vi "数据库存储.vi"(3 "输出簇":T1) -> ()   [LabVIEW 2010]
panel:
  in  "error in (no error)":errorcluster caption="错误输入（无错误）"
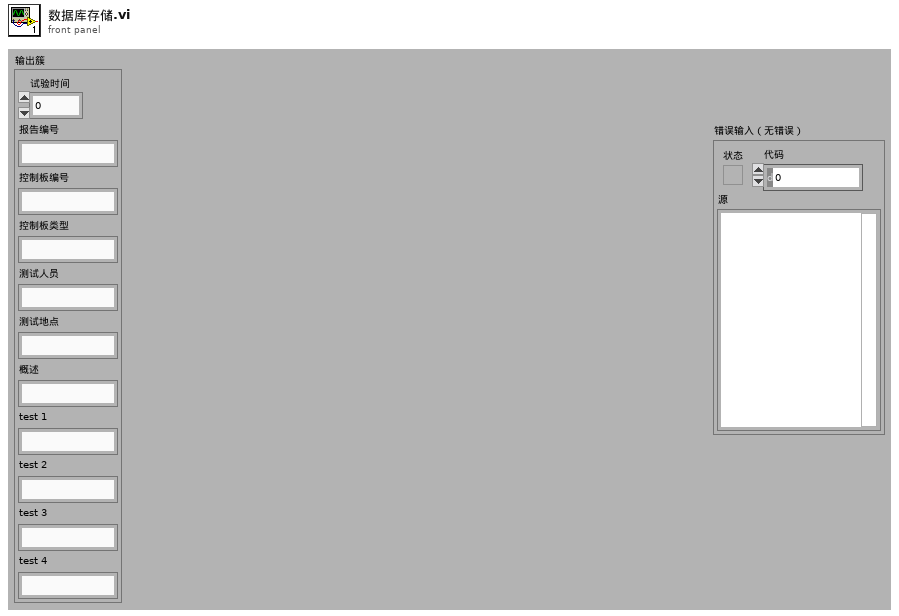
[diagram p1: front panel]
types:
  T1 = cluster{"控制板类型":string, "控制板编号":string, "测试人员":string, "测试地点":string, "报告编号":string, "概述":string, "试验时间":u64, "test 1":string, "test 2":string, "test 3":string, "test 4":string}
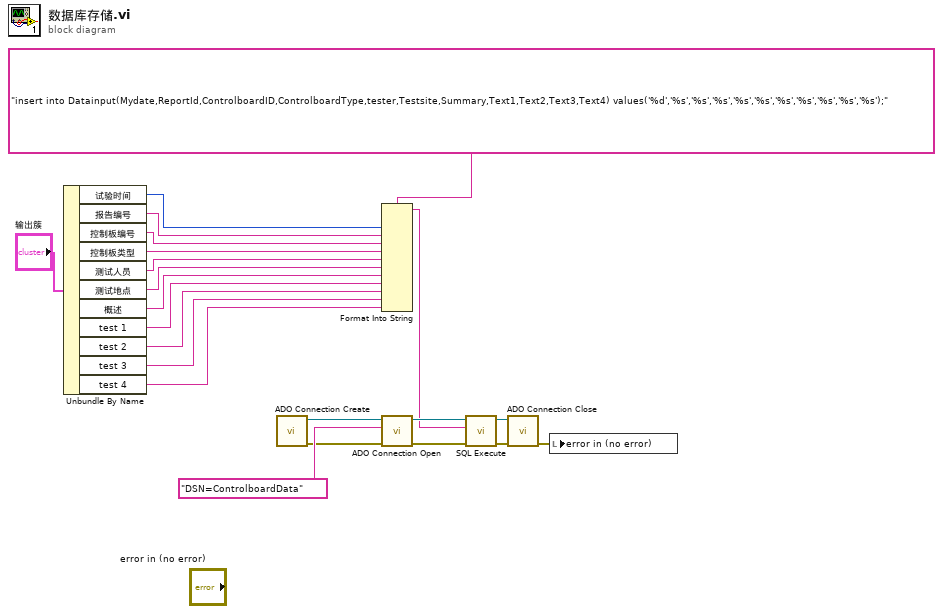
[diagram p0: block diagram]
diagram:
  n1 = Unbundle By Name("输出簇") -> ("试验时间"=w11:u64, "报告编号"=w10:string, "控制板编号"=w9:string, "控制板类型"=w8:string, "测试人员"=w7:string, "测试地点"=w6:string, "概述"=w5:string, "test 1"=w4:string, "test 2"=w3:string, "test 3"=w2:string, "test 4"=w1:string)
  n2 = call "ADO Connection Create.vi"() -> ("error out"=w14:errorcluster, "ADODB._Connection Out"=w13:refnum<k7>)  [unwired: 10 in]
  n3 = Format Into String(format string="insert into Datainput(Mydate,ReportId,ControlboardID,ControlboardType,tester,Testsite,Summary,Text1,Text2,Text3,Text4) values('%d','%s','%s','%s','%s','%s','%s','%s','%s','%s','%s');", w11, w10, w9, w8, w7, w6, w5, w4, w3, w2, w1) -> (resulting string=w12:string)  [unwired: 2 in, 1 out]
  n4 = call "ADO Connection Open.vi"("error in (no error)"=w14, "ConnectionString"="DSN=ControlboardData", "ADODB._Connection In"=w13) -> ("error out"=w17:errorcluster, "ADODB._Connection Out"=w20:refnum<k7>)  [unwired: 7 in]
  n5 = call "SQL Execute.vi"("error in (no error)"=w17, "Command Text"=w12, "ADODB._Connection In"=w20) -> ("error out"=w16:errorcluster, "ADODB._Connection Out"=w19:refnum<k7>)  [unwired: 5 in, 2 out]
  n6 = call "ADO Connection Close.vi"("error in (no error)"=w16, "ADODB._Connection In"=w19) -> ("error out"=w15:errorcluster)  [unwired: 8 in, 1 out]
  n7 = local write "error in (no error)"(w15) -> ()
